vi "Begin.vi"(8 "error in":errorcluster) -> (0 "error out":errorcluster)   [LabVIEW 2019]
doc: "Called before other user functions, this VI is expected to open initial I/O refnums, load in file data, and do all program initialization. Notice that the <B>error out</B> terminal is simply used for data flow. Wiring it to other structures or subVIs ensures that this VI runs first."
uses:
  <vilib>/Rock Robotics/WPI/DriverStation/WPI_DriverStationRobotMode2.ctl
  <vilib>/Rock Robotics/WPI/Joystick/WPI_JoystickDeviceEnum.ctl
  <vilib>/Rock Robotics/SystemInterfaces/AI/FPGA_AIGyroChannel.ctl
  <vilib>/Rock Robotics/SystemInterfaces/DIO/FPGA_DIOPWMChannel.ctl
  <vilib>/Rock Robotics/SystemInterfaces/DIO/FPGA_DIOChannel.ctl
  Robot Global Data.vi
  <vilib>/Rock Robotics/Network Tables/NT Write String Array.vi
  <vilib>/Rock Robotics/WPI/Gyro/WPI_GyroAnalogOpen.vi
  <vilib>/Rock Robotics/WPI/ThirdParty/JAS_Junk/TrajLib/Trajectory_Library.lvlib
panel:
  in  "Tab Control":T1(tab)
  # "Instructions:\nThis should create a path, show the data on the various tabs and optionally write the motor demands and expected results to a file for use on a a robot..\n1) Enter robot data on Robot Data Tab\n2) Define your path definitions.\n3) Define the time increment.  0.020 is chosen since that matches the normal loop time.\n4) Press calculate path.  If a good path was calculated it will be displayed on the Tank Data tab, and the Ready to Execute will indicate execution can begin.\nThe path can be recalculated many times before selecting execute.\n\nTo write to a file.\n5) Select the file name\n6) This example uses \"steps\", sequential numbers for inclusion into a list based autonomous routine.  Including the step number if optional.\n7) This uses command numbers to indicate first, last, and intermediate steps.  This allows some simplification of the execution routine.  It\nalso allows the path to be executed backwards if desired.  The command numbers are changeable.\n8) Press \"Create Command List\".\n\nNotes:\n- PC robot simulataion is disabled in this program.  The code is still there if you want to restore it and try it out.  Use one of the other test programs \nto simulate the path on a PC.\n- The path generation logic doesn't account distribution of speed to the left and right wheels.  As a result the maximum speed can be exceeded.\nIf this happens, but Path Speed > Max light will light and Ready to Execute will not light.  Lower the maximum speed in the Robot Data tab\nand recalulate the path.\n- 2019 playing field size - width: 26 ft 11.25 In = 323.25 in , length: 52 ft 5.25 in = 629.25 in  (I didn't verify this for the 2020 version.)"
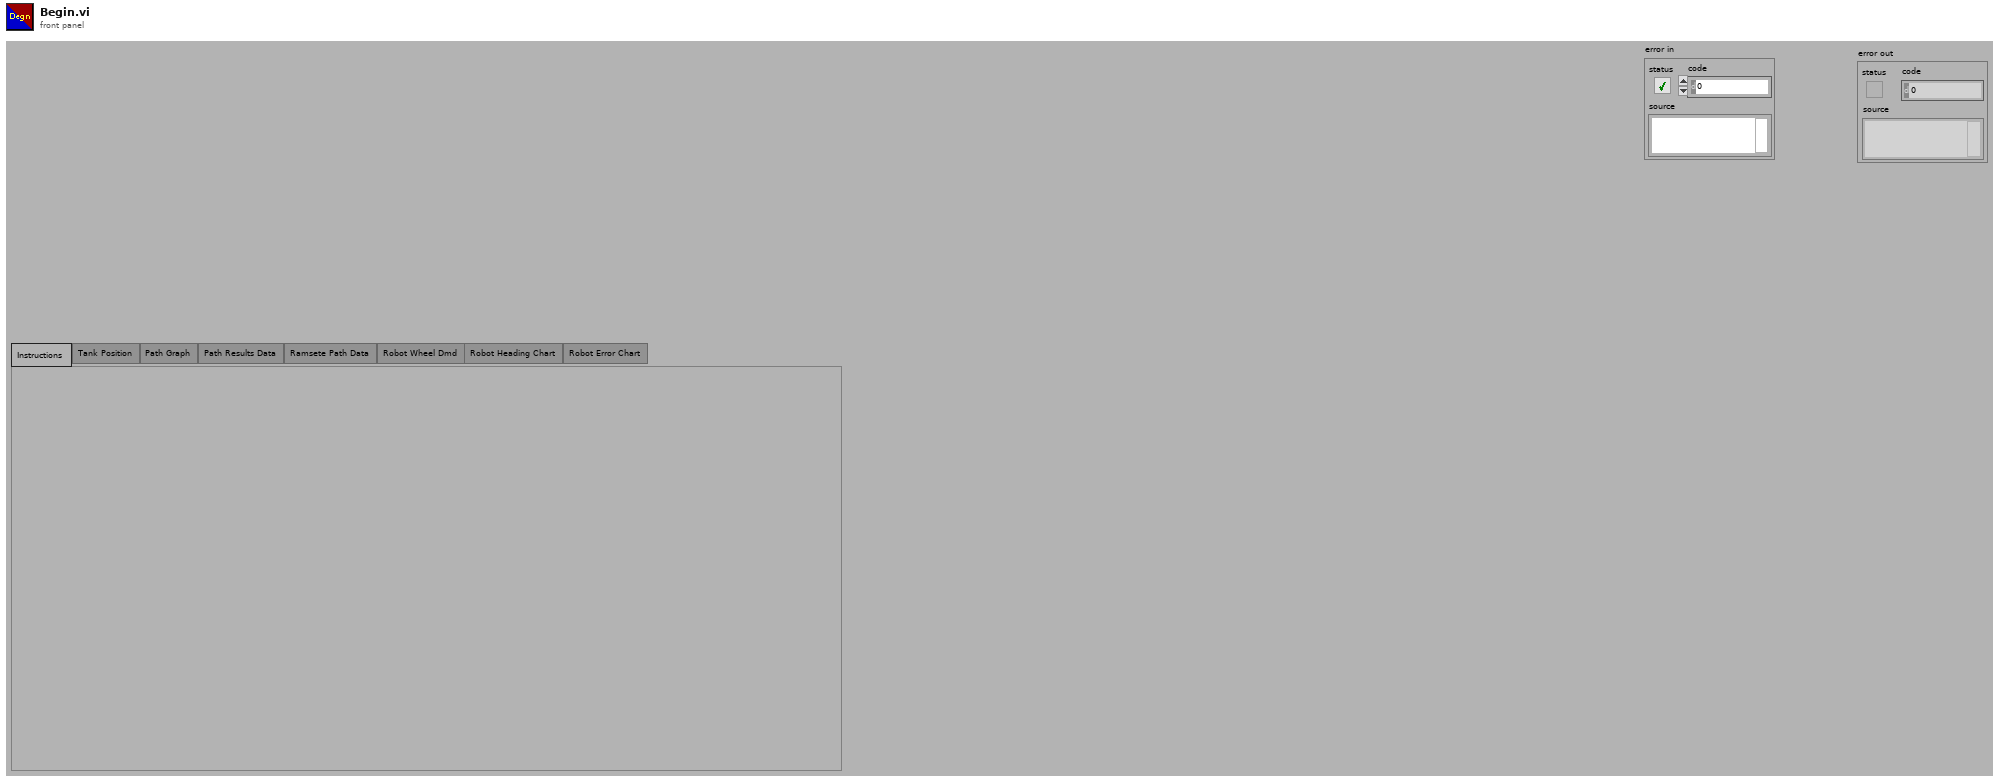
[diagram p1: front panel]
types:
  T1 = enum32{"Instructions", "Tank Position", "Path Graph", "Path Results Data", "Ramsete Path Data", "Robot Wheel Dmd", "Robot Heading Chart", "Robot Error Chart"}
  T2 = typedef "FPGA_DIOChannel.ctl" = enum8{"DIO 0", "DIO 1", "DIO 2", "DIO 3", "DIO 4", "DIO 5", "DIO 6", "DIO 7", "DIO 8", "DIO 9", "DIO MXP 0", "DIO MXP 1", "DIO MXP 2", "DIO MXP 3", "DIO MXP 4", "DIO MXP 5", "DIO MXP 6", "DIO MXP 7", "DIO MXP 8", "DIO MXP 9", "DIO MXP 10", "DIO MXP 11", "DIO MXP 12", "DIO MXP 13", "DIO MXP 14", "DIO MXP 15", "SPI Port CS1", "SPI Port CS2", "SPI Port CS3", "SPI Port MISO", "SPI Port MOSI", "Invalid"}
  T3 = typedef "FPGA_DIOPWMChannel.ctl" = enum8{"PWM 0", "PWM 1", "PWM 2", "PWM 3", "PWM 4", "PWM 5", "PWM 6", "PWM 7", "PWM 8", "PWM 9", "PWM MXP 0", "PWM MXP 1", "PWM MXP 2", "PWM MXP 3", "PWM MXP 4", "PWM MXP 5", "PWM MXP 6", "PWM MXP 7", "PWM MXP 8", "PWM MXP 9", "Invalid"}
  T4 = typedef "FPGA_AIGyroChannel.ctl" = enum8{"AI 0", "AI 1", "Invalid"}
  T5 = typedef "WPI_JoystickDeviceEnum.ctl" = enum16{"USB 0", "USB 1", "USB 2", "USB 3", "USB 4", "USB 5"}
  T6 = typedef "WPI_DriverStationRobotMode2.ctl" = enum16{"Autonomous Disabled", "Autonomous Enabled", "Teleop Disabled", "Teleop Enabled", "Disconnected", "Finish", "Test Disabled", "Test Enabled", "Emergency Stopped"}
  T7 = typedef "WPI_JoystickDevRef.ctl" = cluster{"Device":T5}
  T8 = typedef "WPI_GyroDevRef.ctl" = cluster{"DevStatus":errorcluster, "Analog Channel":T9, "Gain (VoltsPerDegree/Second)":dbl, "Gyro Type":enum16{"Analog", "XRS450"}, "Handle":i32, "SPI Bus":T10, "Device Found":bool, "Sample Rate":dbl, "Calibrate On Open":bool, "Offset":dbl}
  T9 = typedef "FPGA_AIChannel.ctl" = enum8{"AI 0", "AI 1", "AI 2", "AI 3", "AI MXP 0", "AI MXP 1", "AI MXP 2", "AI MXP 3", "Invalid"}
  T10 = typedef "spi_bus.ctl" = enum16{"SPI On-Board, CS0", "SPI On-Board, CS1", "SPI On-Board, CS2", "SPI On-Board, CS3", "SPI MXP", "Invalid"}
  T11 = typedef "Trajectory_Library.lvlib/TRANSLATION2D.ctl" = cluster{"X":dbl, "Y":dbl}
  T12 = typedef "Trajectory_Library.lvlib/ROTATION2D.ctl" = cluster{"VALUE":dbl, "COS":dbl, "SIN":dbl}
  T13 = typedef "Trajectory_Library.lvlib/POSE2D.ctl" = cluster{"TRANSLATION":T11, "ROTATION":T12}
  T14 = typedef "Trajectory_Library.lvlib/SWERVE_DRIVE_ODOMETRY.ctl" = cluster{"POSE":T13, "GyroOffset":T12, "PreviousAngle":T12, "PrevTime":dbl}
  T15 = typedef "Trajectory_Library.lvlib/SWERVE_DRIVE_KINEMATICS.ctl" = cluster{"NumModules":i32, "InverseKinematics":T16, "ForwardKinematics":T16, "Modules":T11[], "PrevCoR":T11}
  T16 = typedef "NI_Matrix.lvlib/RealMatrix.ctl" = dbl[][]
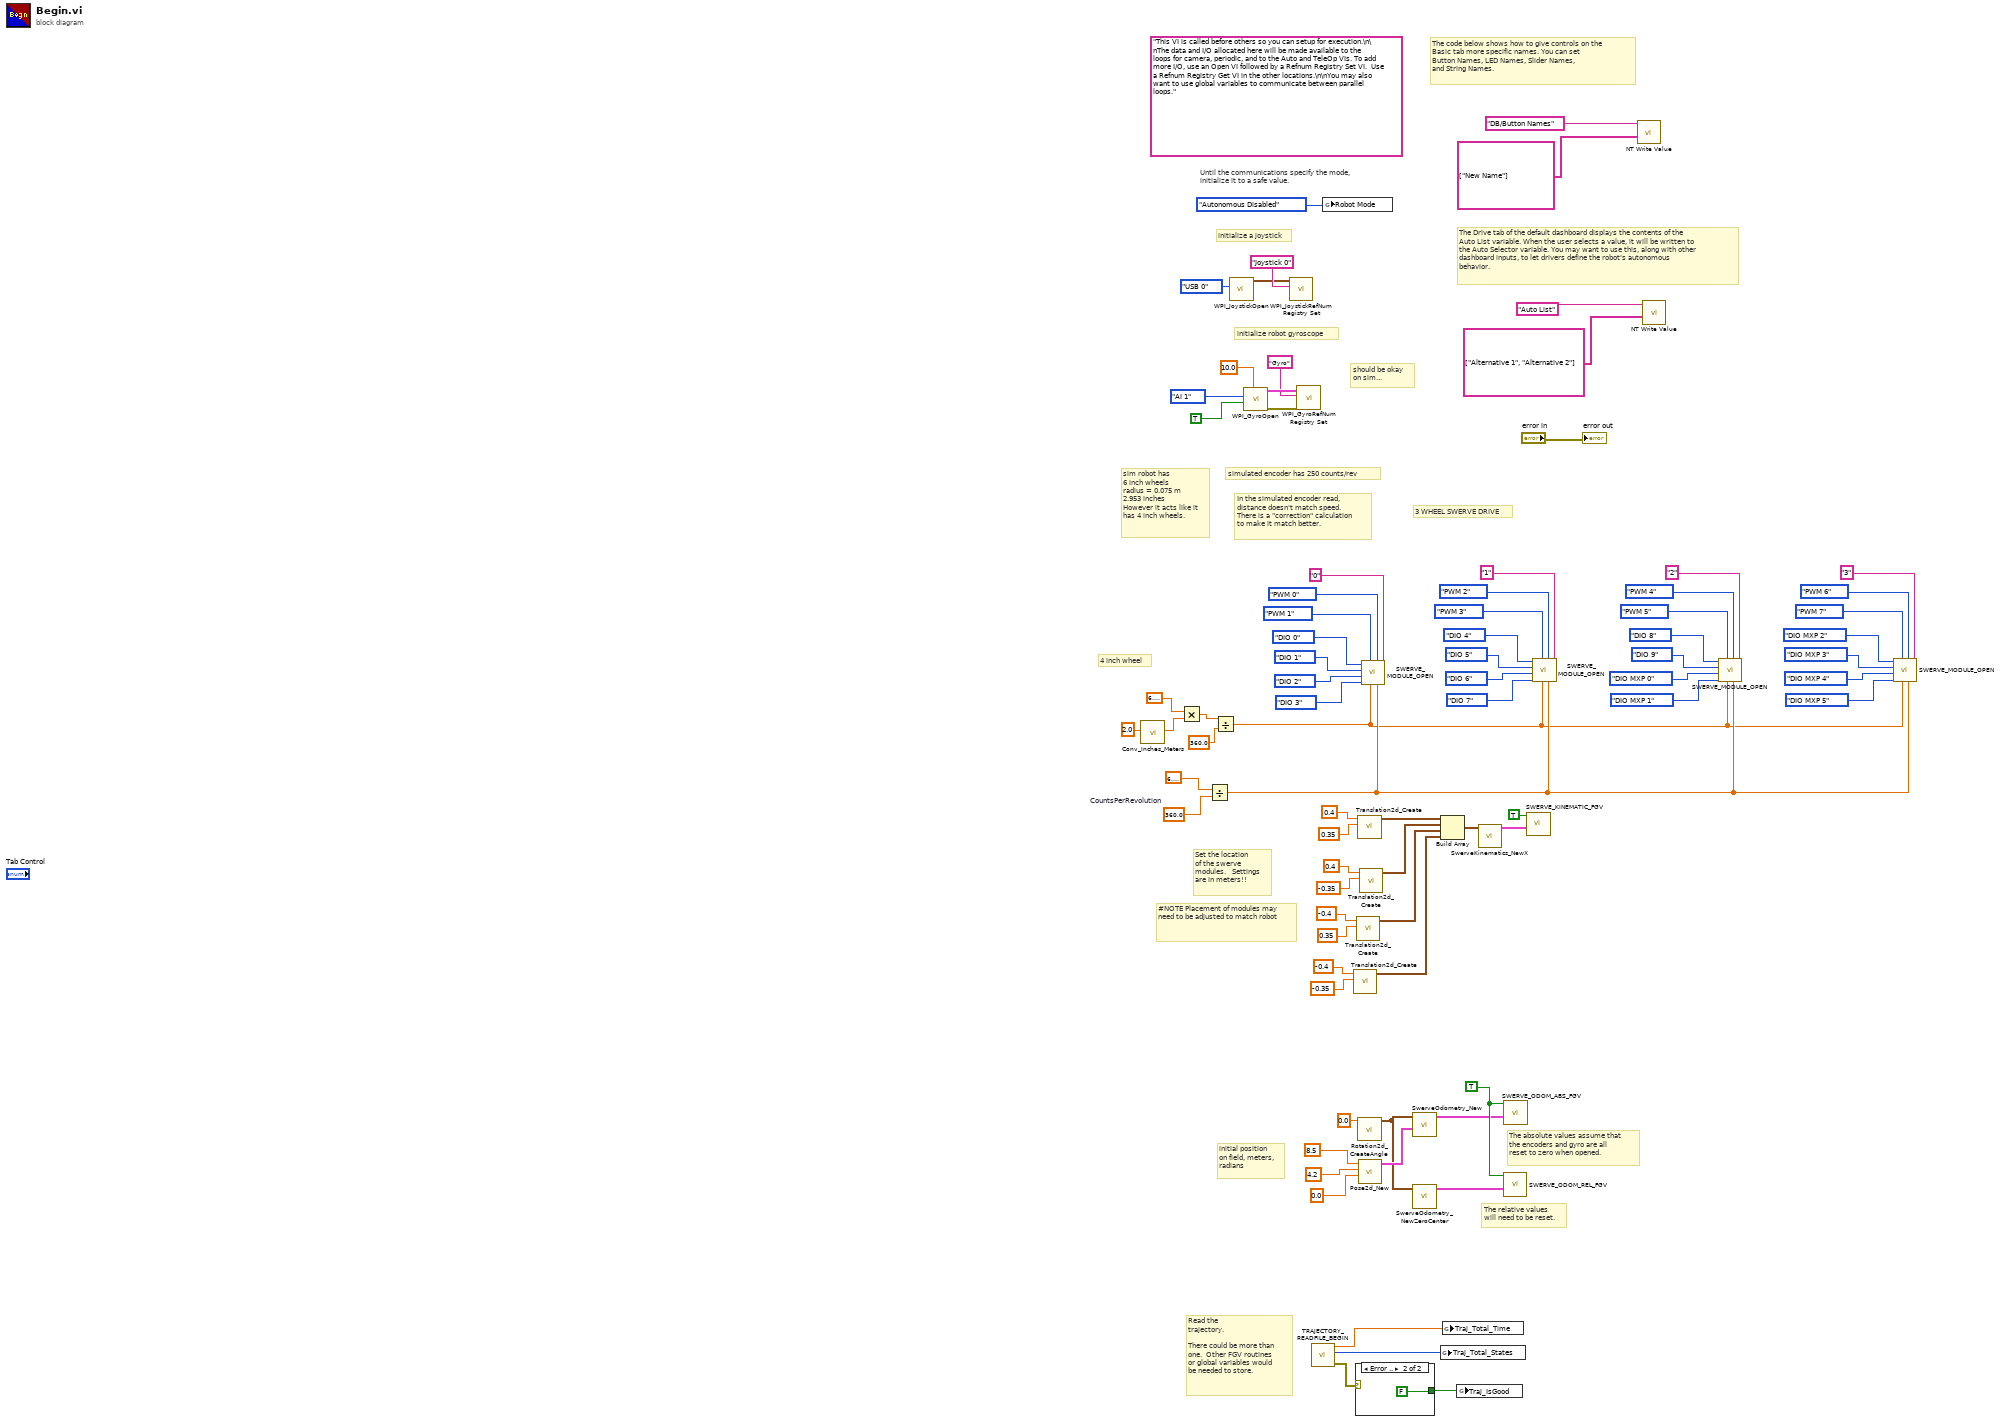
[diagram p0: block diagram]
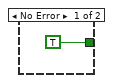
[diagram p2: hidden frame]
diagram:
  w16 = TRUE ("WRITE")
  w50 = 360.0  # CountsPerRevolution
  (unwired) "This VI is called before others so you can setup for execution.\n\nThe data and I/O allocated here will be made available to the loops for camera, periodic, and to the Auto and TeleOp VIs. To add more I/O, use an Open VI followed by a Refnum Registry Set VI.  Use a Refnum Registry Get VI in the other locations.\n\nYou may also want to use global variables to communicate between parallel loops."
  # "#NOTE Placement of modules may need to be adjusted to match robot"
  # "should be okay\non sim..."
  # "The absolute values assume that\nthe encoders and gyro are all\nreset to zero when opened."
  # "The relative values\nwill need to be reset."
  # "initial position\non field, meters,\nradians"
  # "Set the location\nof the swerve \nmodules.   Settings\nare in meters!!"
  # "4 inch wheel"
  # "3 WHEEL SWERVE DRIVE"
  # "initialize robot gyroscope"
  # "Read the\ntrajectory.\n\nThere could be more than\none.  Other FGV routines\nor global variables would\nbe needed to store."
  # "In the simulated encoder read,\ndistance doesn't match speed.\nThere is a \"correction\" calculation\nto make it match better."
  # "simulated encoder has 250 counts/rev"
  # "sim robot has\n6 inch wheels\nradius = 0.075 m\n2.953 inches\nHowever it acts like it\nhas 4 inch wheels."
  # "The Drive tab of the default dashboard displays the contents of the\nAuto List variable. When the user selects a value, it will be written to\nthe Auto Selector variable. You may want to use this, along with other\ndashboard inputs, to let drivers define the robot's autonomous\nbehavior."
  # "The code below shows how to give controls on the\nBasic tab more specific names. You can set\nButton Names, LED Names, Slider Names,\nand String Names."
  # "initialize a joystick"
  # "Until the communications specify the mode,\ninitialize it to a safe value."
  n1 = call <vilib>:"Conv_Inches_Meters.vi"("INCH"=2.0) -> ("Meters"=w22:dbl)  [unwired: 10 in]
  n2 = Multiply(x=6.283185307179586, y=w22) -> (x*y=w70:dbl)
  n3 = Divide(x=6.283185307179586, y=w50) -> (x/y=w5:dbl)
  n4 = Divide(x=w70, y=360.0) -> (x/y=w4:dbl)
  n5 = call <vilib>:"WPI_JoystickOpen.vi"("JoystickDevice"=WPI_JoystickDeviceEnum."USB 0") -> ("JoystickDevRef"=w78:T7)  [unwired: 10 in]
  n6 = call-poly <vilib>:"WPI_GyroOpen.vi"("Calibration Time (s)"=10.0, "Calibrate On Open"=TRUE, "Analog Channel"=FPGA_AIGyroChannel."AI 1") -> ("error out"=w67:errorcluster, "GyroDevRef"=w66:T8)  [unwired: 6 in, 1 out]
  n7 = call <vilib>:"WPI_JoystickRefNum Registry Set.vi"("refnum name"="Joystick 0", "JoystickDevRef"=w78) -> ()  [unwired: 8 in, 2 out]
  n8 = call <vilib>:"WPI_GyroRefNum Registry Set.vi"("error in (no error)"=w67, "refnum name"="Gyro", "GyroDevRef"=w66) -> ()  [unwired: 7 in, 2 out]
  n9 = call "TRAJECTORY_READFILE_BEGIN.vi"() -> ("error out"=w64:errorcluster, "Trajectory Items"=w61:i32, "TotalTImeSecs"=w62:dbl)  [unwired: 9 in]
  n10 = global write "Robot Global Data.vi" "Robot Mode"(WPI_DriverStationRobotMode2."Autonomous Disabled" ("Robot Mode")) -> ()
  n11 = call <vilib>:"Translation2d_Create.vi"("Y"=-0.35, "X"=-0.4) -> ("TRANSLATION"=w1:T11)  [unwired: 9 in]
  n12 = case shown="Error .." w64 {
    tunnel: [TRUE FALSE] -> w63
    frame No Error {
    }
    frame Error {
    }
  }
  n13 = call <vilib>:"Translation2d_Create.vi"("Y"=0.35, "X"=-0.4) -> ("TRANSLATION"=w27:T11)  [unwired: 9 in]
  n14 = call <vilib>:"Translation2d_Create.vi"("Y"=0.35, "X"=0.4) -> ("TRANSLATION"=w29:T11)  [unwired: 9 in]
  n15 = call <vilib>:"Rotation2d_CreateAngle.vi"("Angle"=0.0) -> ("ROTATION"=w14:T12)  [unwired: 10 in]
  n16 = call <vilib>:"Pose2d_New.vi"("Heading"=0.0, "Y"=4.2, "X"=8.5) -> ("out POSe"=w17:T13)  [unwired: 8 in]
  n17 = call <vilib>:"Translation2d_Create.vi"("Y"=-0.35, "X"=0.4) -> ("TRANSLATION"=w28:T11)  [unwired: 9 in]
  n18 = call "SWERVE_MODULE_OPEN.vi"("NameSuffix"="0", "RadiansPerCount"=w5, "Drive PWM Channel"=FPGA_DIOPWMChannel."PWM 0", "DistancePerCount"=w4, "Swerve PWM Channel"=FPGA_DIOPWMChannel."PWM 1", "Swerve B Channel"=FPGA_DIOChannel."DIO 3", "Swerver A Channel"=FPGA_DIOChannel."DIO 2", "Drive B Channel"=FPGA_DIOChannel."DIO 1", "Drive A channel"=FPGA_DIOChannel."DIO 0") -> ()  [unwired: 3 in]
  n19 = call <vilib>:"SwerveOdometry_New.vi"("InitialPose"=w17, "gyroAngle"=w14) -> ("SWERVE_DRIVE_ODOMETRY"=w15:T14)  [unwired: 9 in]
  n20 = call <vilib>:"SwerveOdometry_NewZeroCenter.vi"("gyroAngle"=w14) -> ("SWERVE_DRIVE_ODOMETRY"=w13:T14)  [unwired: 10 in]
  n21 = global write "Robot Global Data.vi" "Traj_Total_States"(w61) -> ()
  n22 = Build Array(w29, w28, w27, w1) -> (w26:T11[])
  n23 = global write "Robot Global Data.vi" "Traj_Total_Time"(w62) -> ()
  n24 = global write "Robot Global Data.vi" "Traj_IsGood"(w63) -> ()
  n25 = call <vilib>:"SwerveKinematics_NewX.vi"("Wheels"=w26) -> ("SWERVE_DRIVE_KINEMATICS"=w24:T15)  [unwired: 10 in]
  n26 = call "SWERVE_ODOM_REL_FGV.vi"("in SWERVE_DRIVE_ODOMETRY"=w13, "WRITE"=w16) -> ()  [unwired: 9 in, 1 out]
  n27 = call "SWERVE_ODOM_ABS_FGV.vi"("in SWERVE_DRIVE_ODOMETRY"=w15, "WRITE"=w16) -> ()  [unwired: 9 in, 1 out]
  n28 = call "SWERVE_KINEMATIC_FGV.vi"("in SWERVE_DRIVE_KINEMATICS"=w24, "WRITE"=TRUE) -> ()  [unwired: 9 in, 1 out]
  n29 = call "SWERVE_MODULE_OPEN.vi"("NameSuffix"="1", "RadiansPerCount"=w5, "Drive PWM Channel"=FPGA_DIOPWMChannel."PWM 2", "DistancePerCount"=w4, "Swerve PWM Channel"=FPGA_DIOPWMChannel."PWM 3", "Swerve B Channel"=FPGA_DIOChannel."DIO 7", "Swerver A Channel"=FPGA_DIOChannel."DIO 6", "Drive B Channel"=FPGA_DIOChannel."DIO 5", "Drive A channel"=FPGA_DIOChannel."DIO 4") -> ()  [unwired: 3 in]
  n30 = call-poly <vilib>:"NT Write Value.vi"("String Array"=string[] ["New Name"], "Name"="DB/Button Names") -> ()  [unwired: 9 in, 1 out]
  n31 = call-poly <vilib>:"NT Write Value.vi"("String Array"=string[] ["Alternative 1", "Alternative 2"], "Name"="Auto List") -> ()  [unwired: 9 in, 1 out]
  n32 = call "SWERVE_MODULE_OPEN.vi"("NameSuffix"="2", "RadiansPerCount"=w5, "Drive PWM Channel"=FPGA_DIOPWMChannel."PWM 4", "DistancePerCount"=w4, "Swerve PWM Channel"=FPGA_DIOPWMChannel."PWM 5", "Swerve B Channel"=FPGA_DIOChannel."DIO MXP 1", "Swerver A Channel"=FPGA_DIOChannel."DIO MXP 0", "Drive B Channel"=FPGA_DIOChannel."DIO 9", "Drive A channel"=FPGA_DIOChannel."DIO 8") -> ()  [unwired: 3 in]
  n33 = call "SWERVE_MODULE_OPEN.vi"("NameSuffix"="3", "RadiansPerCount"=w5, "Drive PWM Channel"=FPGA_DIOPWMChannel."PWM 6", "DistancePerCount"=w4, "Swerve PWM Channel"=FPGA_DIOPWMChannel."PWM 7", "Swerve B Channel"=FPGA_DIOChannel."DIO MXP 5", "Swerver A Channel"=FPGA_DIOChannel."DIO MXP 4", "Drive B Channel"=FPGA_DIOChannel."DIO MXP 3", "Drive A channel"=FPGA_DIOChannel."DIO MXP 2") -> ()  [unwired: 3 in]
  "error out" <- "error in"
